vi "DisableControls.vi"(8 "Error In":errorcluster, 10 "Lock Controls (F)":bool, 11 "Reference To Disable":refnum<vi>[](array[refnum])) -> (0 "Error Out":errorcluster)   [LabVIEW 2018]
doc: "This VI disables and greys out the controls."
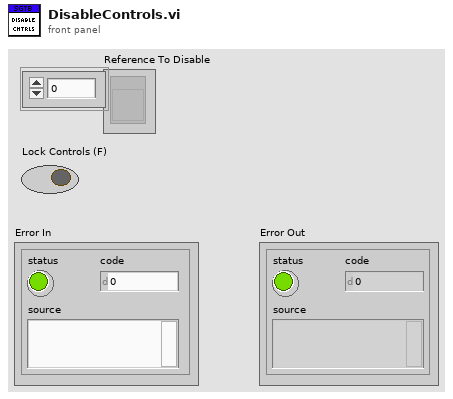
[diagram p1: front panel]
types:
  T1 = enum8{"Enabled", "Disabled", "Disabled and Grayed Out"}
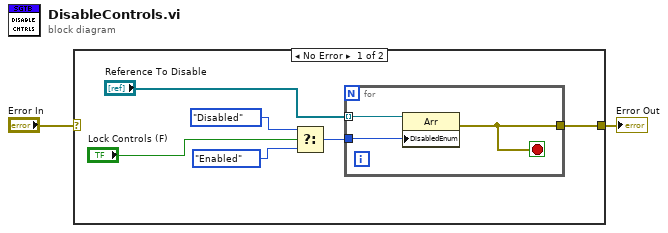
[diagram p0: block diagram]
diagram:
  n1 = case shown="No Error" "Error In" {
    selector: "Error In" -> [_ w12]
    tunnel: [w8 w12] -> w1
    frame No Error {
      n2 = Select(t=T1."Disabled" ("Disabled"), s="Lock Controls (F)", f=T1."Enabled" ("Disabled")) -> (s? t:f=w4:T1)
      n3 = for {
        tunnel: [w11] -> w8
        tunnel: w4 -> [w10]
        tunnel: "Reference To Disable" -> [w9] mode=indexing
        stop <- w11 stop-if-true
        n4 = property on="Property Node" class="Arr"(reference=w9, "DisabledEnum"=w10) -> (error out=w11:errorcluster)  [unwired: 1 in, 1 out]
      }
    }
    frame Error {
    }
  }
  "Error Out" <- w1
